vi "Add Battery Switch Card From Table.vi"(8 "error in (no error)":errorcluster, 10 "Card Position":T1={"Rack #"=0, "Slot #"=1} {"Slot #" max=15}, 11 "Node Ptr":u64 format="%.0x") -> (0 "error out":errorcluster)   [LabVIEW 2014, in "SLSC configuration System Explorer.lvlib"]
uses:
  SLSC configuration System Explorer.lvlib
  Type Defs/Card Position.ctl
  Shared/SPI Utility/Slot #.ctl
  Shared/Constants.vi
  Shared/SLSC configuration Shared.lvlib
panel:
  in  "Tag":string
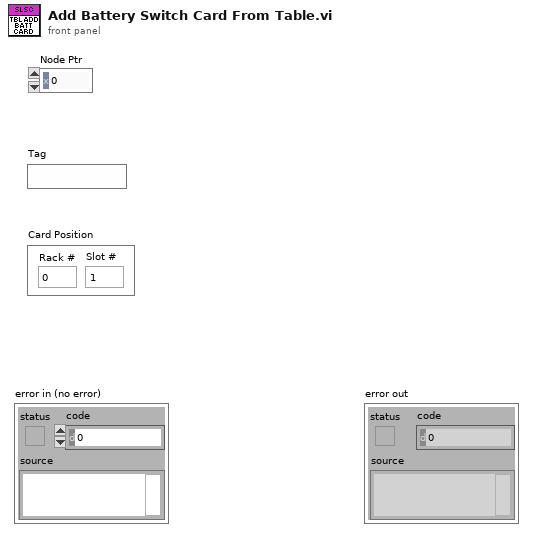
[diagram p1: front panel]
types:
  T1 = typedef "SLSC configuration Shared.lvlib/Card Position.ctl" = cluster{"Rack #":u8, "Slot #":T2}
  T2 = typedef "SLSC configuration Shared.lvlib/Slot #.ctl" = u8
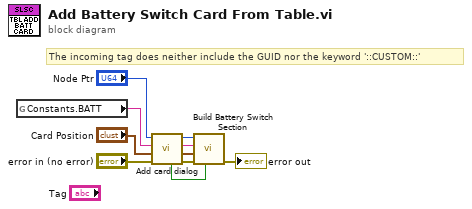
[diagram p0: block diagram]
diagram:
  # "The incoming tag does neither include the GUID nor the keyword '::CUSTOM::'"
  n1 = global read "Constants.vi" "Constants.BATT"() -> (w8:string)
  n2 = call "Add card dialog.vi"("error in (no error)"="error in (no error)", "Card Position"="Card Position", "Card Type in"=w8, "Node Ptr"="Node Ptr") -> ("error out"=w7:errorcluster, "Card Position out"=w5:T1, "Name out"=w3:string, "Node Ptr out"=w2:u64, "Cancelled?"=w4:bool)  [unwired: 3 in]
  n3 = call "Build Battery Switch Section.vi"("Cancelled?"=w4, "error in (no error)"=w7, "Card Position in"=w5, "Name in"=w3, "Node Ptr in"=w2) -> ("error out"=→"error out":errorcluster)  [unwired: 6 in]
